vi "WSVCAP SHL Host TL Tester - Dual Board.vi"   [LabVIEW 2012]
uses:
  Type Defs/WSVCAP SHL I2C FPGA Enum.ctl
types:
  T1 = typedef "WSVCAP SHL I2C FPGA Enum.ctl" = enum16{"RIO0", "RIO1"}
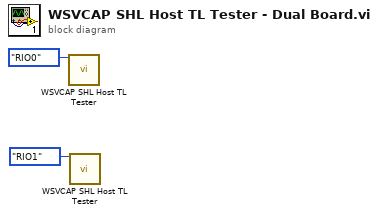
[diagram p0: block diagram]
diagram:
  n1 = call "WSVCAP SHL Host TL Tester.vi"("FPGA"=WSVCAP_SHL_I2C_FPGA_Enum."RIO0") -> ()  [unwired: 15 in]
  n2 = call "WSVCAP SHL Host TL Tester.vi"("FPGA"=WSVCAP_SHL_I2C_FPGA_Enum."RIO1") -> ()  [unwired: 15 in]
